vi "Read new experimental header template.vi"() -> ()   [LabVIEW 2017]
uses:
  <vilib>/Utility/config.llb/Read Key (String).vi
  <vilib>/Utility/config.llb/NI_LVConfig.lvlib
panel:
  out "Array":string[][](array[string])
  out "error out":errorcluster
  in  "configuration file path":path
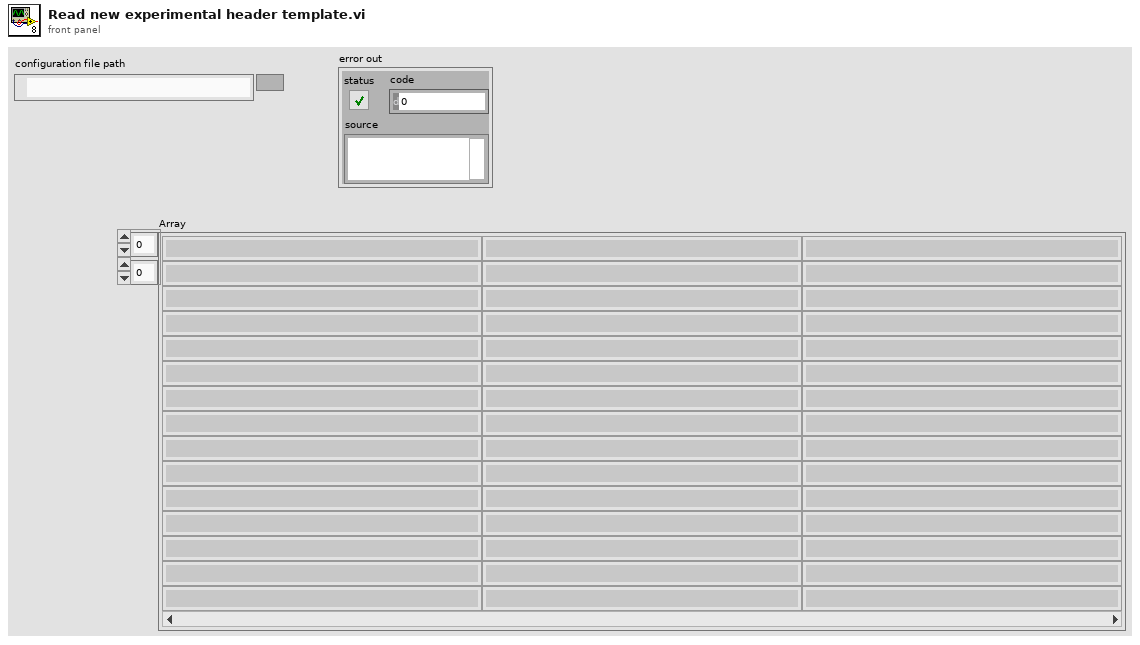
[diagram p1: front panel]
types:
  T1 = typedef "NI_LVConfig.lvlib/Config Data RefNum.ctl" = refnum<k1>
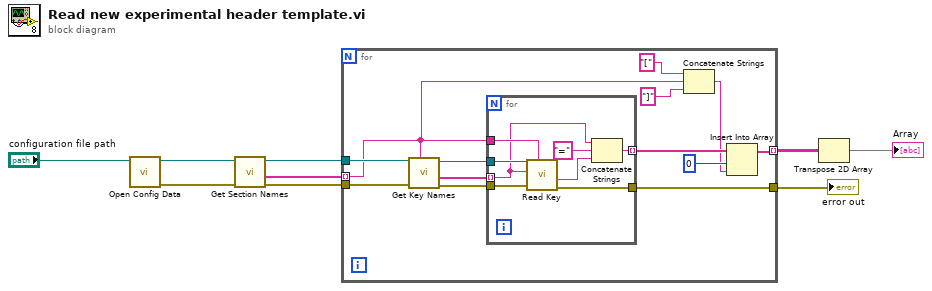
[diagram p0: block diagram]
diagram:
  n1 = call <vilib>:"Open Config Data.vi"("configuration file path"="configuration file path") -> ("error out"=w7:errorcluster, "refnum"=w8:T1)  [unwired: 8 in, 1 out]
  n2 = call <vilib>:"Get Section Names.vi"("error in (no error)"=w7, "refnum"=w8) -> ("error out"=w4:errorcluster, "section names"=w6:string[], "refnum out"=w5:T1)  [unwired: 7 in]
  n3 = for {
    tunnel: w6 -> [w10] mode=indexing
    tunnel: w5 -> [w22]
    tunnel: w4 -> [w19]
    tunnel: [w17] -> w3
    tunnel: [w15] -> w2 mode=indexing
    n4 = call <vilib>:"Get Key Names.vi"("section"=w10, "error in (no error)"=w19, "refnum"=w22) -> ("error out"=w18:errorcluster, "key names"=w21:string[], "refnum out"=w20:T1)  [unwired: 5 in, 1 out]
    n5 = for {
      tunnel: w21 -> [w23] mode=indexing
      tunnel: w20 -> [w30]
      tunnel: w18 -> [w29]
      tunnel: [w28] -> w17
      tunnel: [w25] -> w16 mode=indexing
      tunnel: w10 -> [w24]
      n6 = call-poly <vilib>:"Read Key.vi"("section"=w24, "error in (no error)"=w29, "key"=w23, "refnum"=w30) -> ("error out"=w28:errorcluster, "value"=w26:string)  [unwired: 4 in, 2 out]
      n7 = Concatenate Strings(w23, "=" ("string"), w26) -> (w25:string)
    }
    n8 = Concatenate Strings("[", w10, "]" ("string")) -> (w11:string)
    n9 = Insert Into Array(array=w16, index=0, new element=w11) -> (w15:string[])
  }
  "error out" <- w3
  n10 = Transpose 2D Array(2D array=w2) -> (transposed array=→"Array":string[][])
